vi "FABR-Update SCL.vi"(0 "Runtime in":T2, 7 "SCL in":cluster{T1[]}[](array[cluster]), 11 "error in (no error)":errorcluster) -> (4 "Runtime out":T2, 8 "SCL out":cluster{T1[]}[](array[cluster]), 10 "finished":bool, 15 "error out":errorcluster)   [LabVIEW 2020]
uses:
  Typedefs/FABR-Runtime Data.ctl
  Typedefs/FABR-Stimulus Ticket.ctl
  Typedefs/FABR-Order.ctl
  Typedefs/FABR-Stimulus Condition.ctl
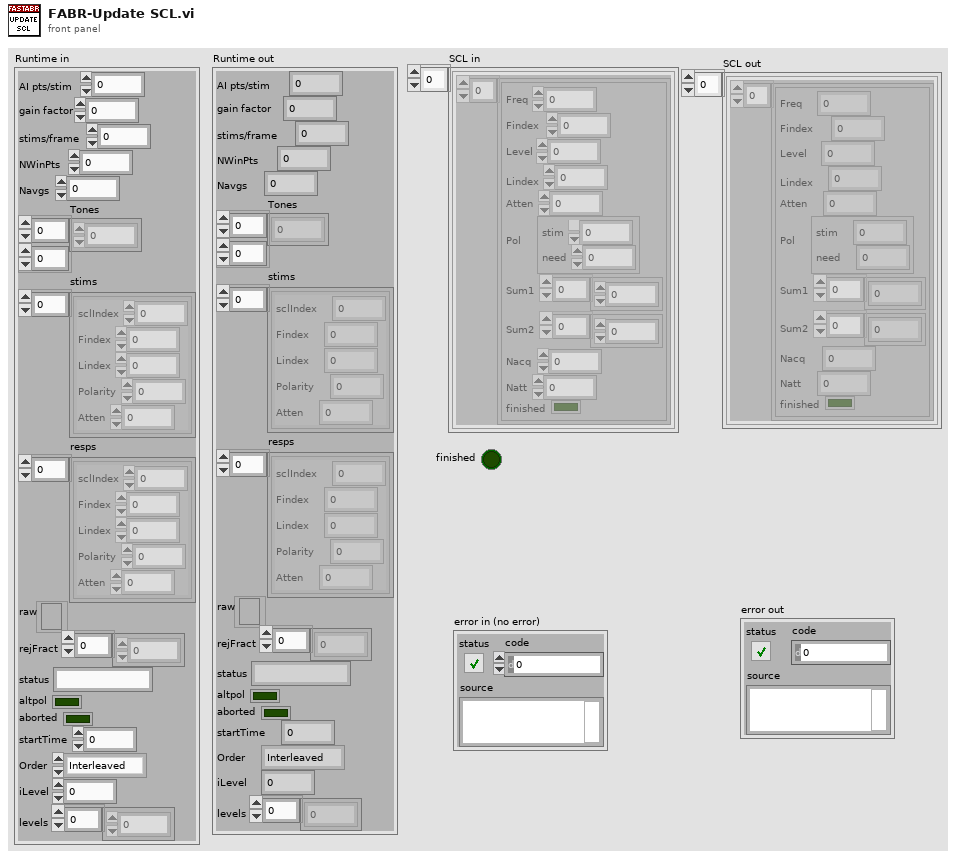
[diagram p1: front panel]
types:
  T1 = typedef "FABR-Stimulus Condition.ctl" = cluster{"Freq":dbl, "Findex":i32, "Level":dbl, "Lindex":i32, "Atten":dbl, "Pol":cluster{"stim":i32, "need":i32}, "Sum1":dbl[], "Sum2":dbl[], "Nacq":i32, "Natt":i32, "finished":bool}
  T2 = typedef "FABR-Runtime Data.ctl" = cluster{"AI pts/stim":i32, "gain factor":dbl, "stims/frame":i32, "NWinPts":i32, "Navgs":i32, "Tones":dbl[][], "stims":T3[], "resps":T3[], "raw":refnum<file>, "rejFract":dbl[], "status":string, "altpol":bool, "aborted":bool, "startTime":dbl, "Order":T4, "iLevel":i32, "levels":dbl[]}
  T3 = typedef "FABR-Stimulus Ticket.ctl" = cluster{"sclIndex":i32, "Findex":i32, "Lindex":i32, "Polarity":i32, "Atten":dbl}
  T4 = typedef "FABR-Order.ctl" = enum16{"Interleaved", "Stepped level"}
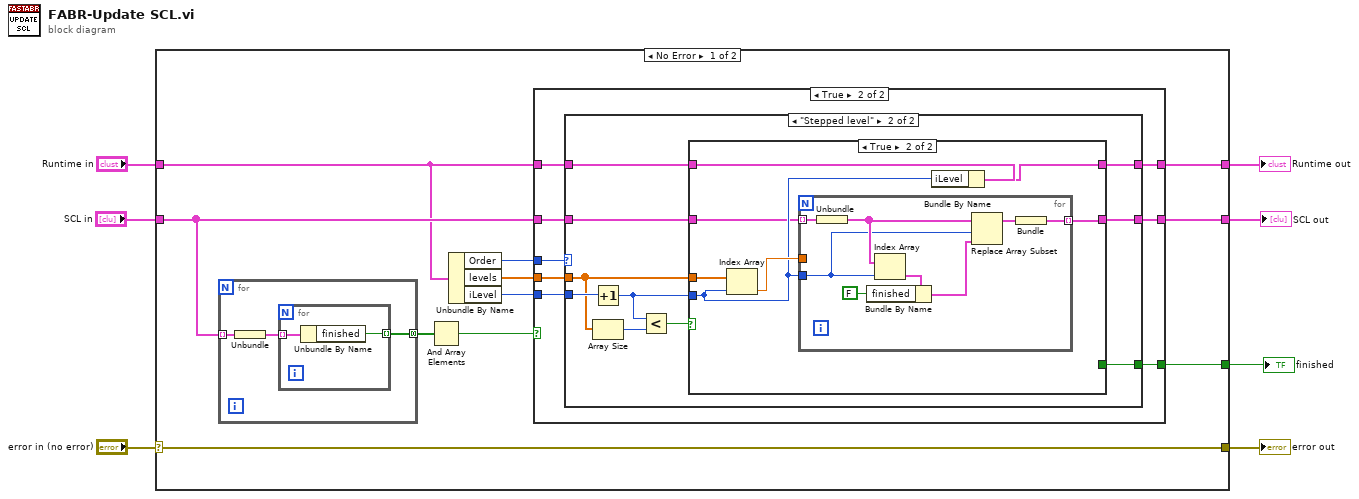
[diagram p0: block diagram]
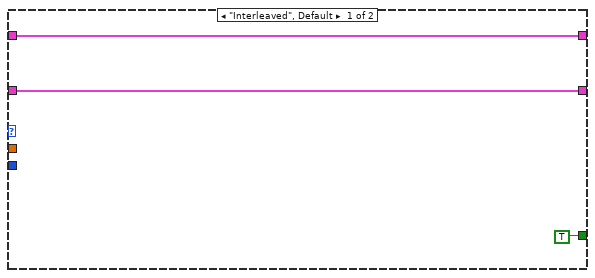
[diagram p3: hidden frame]
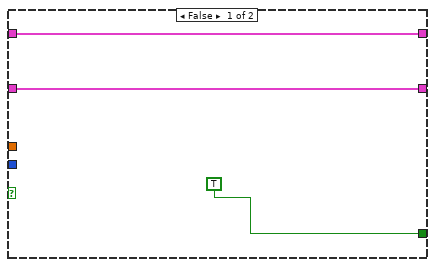
[diagram p4: hidden frame]
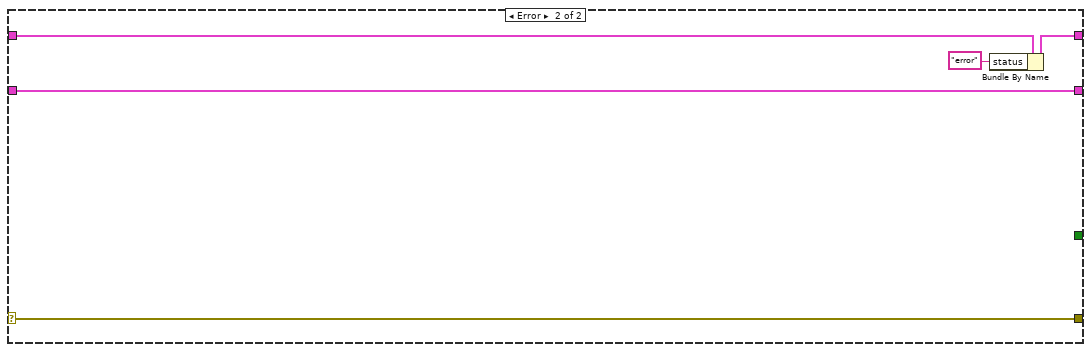
[diagram p5: hidden frame]
diagram:
  n1 = case shown="No Error" "error in (no error)" {
    selector: "error in (no error)" -> [w17 w69]
    tunnel: [w17 w69] -> w6
    tunnel: "SCL in" -> [w13 w65]
    tunnel: [w14 _] -> w4
    tunnel: "Runtime in" -> [w8 w68]
    tunnel: [w12 w67] -> w2
    tunnel: [w11 w65] -> w1
    frame No Error {
      n2 = for {
        tunnel: w13 -> [w62] mode=indexing
        tunnel: [w60] -> w18 mode=concatenating
        # "Count remaining levels by frequency"
        n3 = Unbundle(w62) -> (w61:T1[])
        n4 = for {
          tunnel: w61 -> [w64] mode=indexing
          tunnel: [w63] -> w60 mode=indexing
          n5 = Unbundle By Name(w64) -> ("finished"=w63:bool)
        }
      }
      n6 = And Array Elements(Boolean array=w18) -> (logical AND=w16:bool)
      n7 = Unbundle By Name(w8) -> ("Order"=w15:T4, "levels"=w10:dbl[], "iLevel"=w9:i32)
      n8 = case shown="True" w16 {
        tunnel: w15 -> [_ w21]
        tunnel: [_ w28] -> w14
        tunnel: w8 -> [w20 w27]
        tunnel: w13 -> [w19 w25]
        tunnel: [w20 w26] -> w12
        tunnel: [w19 w24] -> w11
        tunnel: w10 -> [_ w23]
        tunnel: w9 -> [_ w22]
        frame False {
        }
        frame True {
          n9 = case shown="\"Stepped level\"" w21 {
            tunnel: [TRUE w33] -> w28
            tunnel: w27 -> [w30 w38]
            tunnel: [w30 w36] -> w26
            tunnel: w25 -> [w29 w34]
            tunnel: [w29 w35] -> w24
            tunnel: w23 -> [_ w32]
            tunnel: w22 -> [_ w41]
            frame "Interleaved", Default {
            }
            frame "Stepped level" {
              n10 = Increment(x=w41) -> (x+1=w37:i32)
              n11 = Array Size(array=w32) -> (size(s)=w40:i32)
              n12 = Less?(x=w37, y=w40) -> (x < y?=w39:bool)
              n13 = case shown="True" w39 {
                tunnel: w32 -> [_ w49]
                tunnel: w38 -> [w44 w51]
                tunnel: w37 -> [_ w47]
                tunnel: [w44 w50] -> w36
                tunnel: [w43 w45] -> w35
                tunnel: w34 -> [w43 w46]
                tunnel: [TRUE _] -> w33
                frame False {
                }
                frame True {
                  n14 = Index Array(array=w49, index=w47) -> (element=w48:dbl)
                  n15 = for {
                    tunnel: w46 -> [w59] mode=indexing
                    tunnel: w48 -> [_]
                    tunnel: w47 -> [w54]
                    tunnel: [w58] -> w45 mode=indexing
                    n16 = Unbundle(w59) -> (w55:T1[])
                    n17 = Index Array(array=w55, index=w54) -> (element=w57:T1)
                    n18 = Bundle By Name(cluster=w57, "finished"=FALSE) -> (w53:T1)
                    n19 = Replace Array Subset(array=w55, new element=w53, index=w54) -> (w56:T1[])
                    n20 = Bundle(w56) -> (w58:cluster{T1[]})  [unwired: 1 in]
                  }
                  n21 = Bundle By Name(cluster=w51, "iLevel"=w47) -> (w50:T2)
                }
              }
            }
          }
        }
      }
    }
    frame Error {
      n22 = Bundle By Name(cluster=w68, "status"="error") -> (w67:T2)
    }
  }
  "finished" <- w4
  "error out" <- w6
  "Runtime out" <- w2
  "SCL out" <- w1
